vi "updateCategoryAmount.vi"(8 "error in (no error)":errorcluster, 10 "Category.lvclass":refnum<class "Category.lvclass">, 11 "Account History in":refnum<class "Account History.lvclass">) -> (0 "error out":errorcluster, 3 "Account History out":refnum<class "Account History.lvclass">)   [LabVIEW 2020, in "Account History.lvclass"]
uses:
  Account History.lvclass
  Category/Category.lvclass
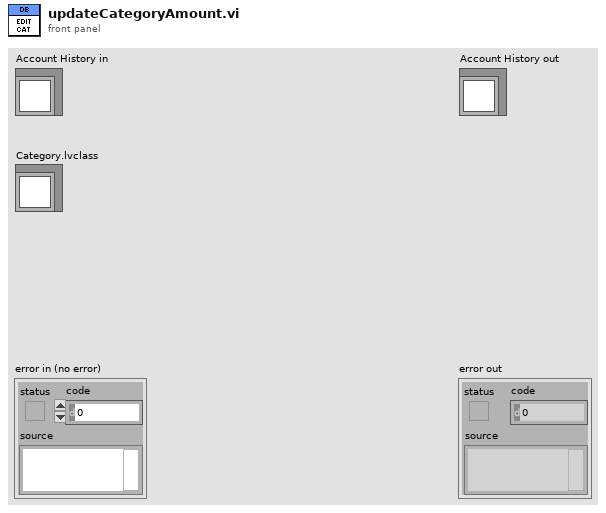
[diagram p1: front panel]
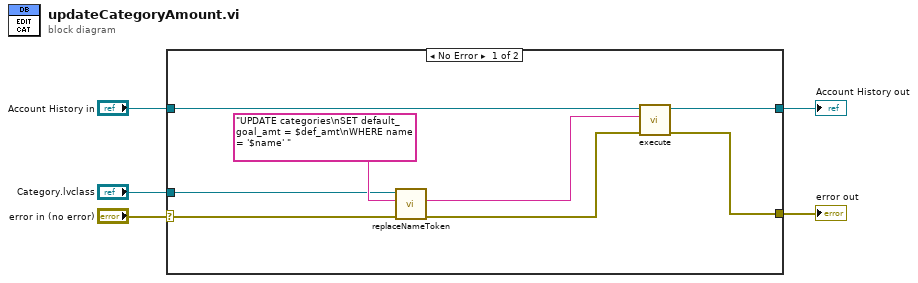
[diagram p0: block diagram]
diagram:
  n1 = case shown="No Error" "error in (no error)" {
    selector: "error in (no error)" -> [w9 w15]
    tunnel: [w11 w15] -> w4
    tunnel: [w12 w14] -> w2
    tunnel: "Account History in" -> [w13 w14]
    tunnel: "Category.lvclass" -> [w8 _]
    frame No Error {
      n2 = call "replaceNameToken.vi"("error in (no error)"=w9, "Query In"="UPDATE categories\nSET default_goal_amt = $def_amt\nWHERE name = '$name' ", "Category in"=w8) -> ("error out"=w7:errorcluster, "Query Out"=w6:string)  [unwired: 6 in, 1 out]
      n3 = call "execute.vi"("error in (no error)"=w7, "SQL query"=w6, "Database in"=w13) -> ("error out"=w11:errorcluster, "Database out"=w12:refnum<class "Account History.lvclass">)  [unwired: 7 in]
    }
    frame Error {
    }
  }
  "error out" <- w4
  "Account History out" <- w2
